vi "AlmostEqual_Rel.vi"(5 "X":dbl format="%_20f", 7 "Tolerance (0.01)":dbl=0.009999999776482582, 9 "Y":dbl format="%_20f") -> (8 "X = Y +/- Tolerance*max(X,Y)?":bool)   [LabVIEW 2020]
doc: "Determines if two single precision numbers are almost equal to eachother.\nTolerance parameter is the maximum relative error between the two numbers. \n\nNotes:\n- Use this function for arbitrarily input values. Tolerance scales relative to input values.\n- Comparison to NaN will always return false.\n- Comparison to +/- Inf will always return false.\n\nSource: http://randomascii.wordpress.com/2012/02/25/comparing-floating-point-numbers-2012-edition/"
panel:
  # "Determines if two single precision numbers are almost equal to eachother.\nTolerance parameter is the maximum relative error between the two numbers. \n\nNotes:\n- Use this function for arbitrarily input values. Tolerance scales relative to input values.\n- Comparison to NaN will always return false.\n- Comparison to +/- Inf will always return false."
  # "Source: http://randomascii.wordpress.com/2012/02/25/comparing-floating-point-numbers-2012-edition/"
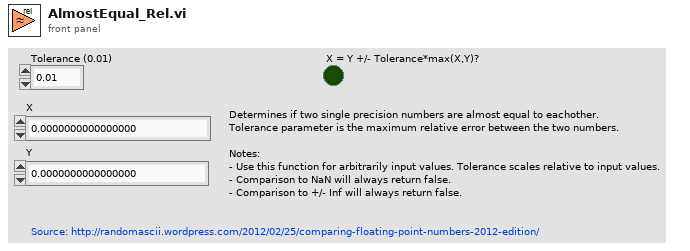
[diagram p1: front panel]
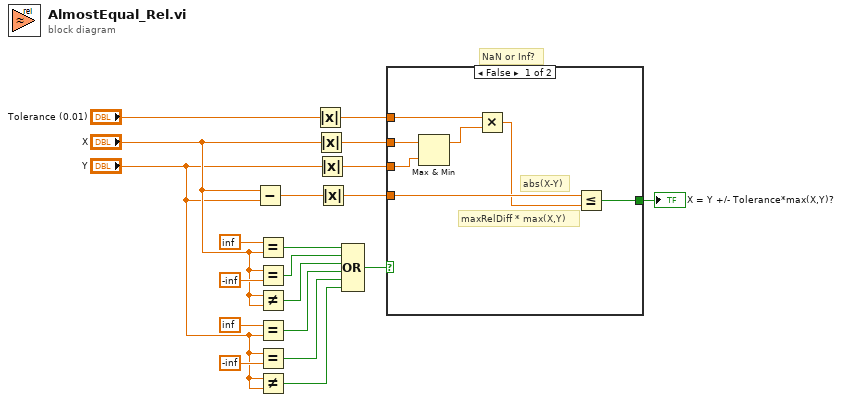
[diagram p0: block diagram]
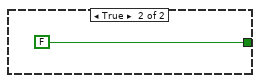
[diagram p2: hidden frame]
diagram:
  # "NaN or Inf?"
  n1 = Subtract(x="X", y="Y") -> (x-y=w16:dbl)
  n2 = Equal?(x=sgl inf, y="X") -> (x = y?=w6:bool)
  n3 = Equal?(x="X", y=sgl -inf) -> (x = y?=w5:bool)
  n4 = Not Equal?(x="X", y="X") -> (x != y?=w4:bool)
  n5 = Equal?(x=sgl inf, y="Y") -> (x = y?=w3:bool)
  n6 = Equal?(x="Y", y=sgl -inf) -> (x = y?=w2:bool)
  n7 = Not Equal?(x="Y", y="Y") -> (x != y?=w1:bool)
  n8 = Absolute Value(x="Tolerance (0.01)") -> (abs(x)=w17:dbl)
  n9 = Absolute Value(x="X") -> (abs(x)=w14:dbl)
  n10 = Absolute Value(x="Y") -> (abs(x)=w13:dbl)
  n11 = Absolute Value(x=w16) -> (abs(x)=w15:dbl)
  n12 = Compound Arithmetic op=OR(w6, w5, w4, w3, w2, w1) -> (w19:bool)
  n13 = case shown="False" w19 {
    tunnel: w17 -> [w23 _]
    tunnel: [w27 FALSE] -> w20
    tunnel: w15 -> [w22 _]
    tunnel: w14 -> [w26 _]
    tunnel: w13 -> [w25 _]
    frame False {
      # "abs(X-Y)"
      # "maxRelDiff * max(X,Y)"
      n14 = Max & Min(x=w26, y=w25) -> (max(x,y)=w24:dbl)  [unwired: 1 out]
      n15 = Multiply(x=w23, y=w24) -> (x*y=w21:dbl)
      n16 = Less Or Equal?(x=w22, y=w21) -> (x <= y?=w27:bool)
    }
    frame True {
    }
  }
  "X = Y +/- Tolerance*max(X,Y)?" <- w20
